vi "OCTavion_ScanControl_Host.vi"() -> ()   [LabVIEW 2016]
uses:
  <vilib>/FPGAPlugInAG/PCIe-7851R/niLvFpga_Open_PCIe-7851R.vi
  <vilib>/rvi/interface/common/dynamic/niFpgaDynamicAddResources.vi
  <vilib>/Utility/error.llb/Error Cluster From Error Code.vi
  <vilib>/rvi/errors/niLvFpgaAdjustHostInterfaceError.vi
  <vilib>/FPGAPlugInAG/Dynamic/niLvFpga_Close_Dynamic.vi
  <vilib>/rvi/interface/nirviOpenFPGA/nirviOpenFPGA.xnode
  FPGA/FPGA Bitfiles/OCTavionScanCont_FPGATarget_OCTavionScanCont_mQLUXe6JE5s.lvbitx
  <vilib>/rvi/interface/nirviReadWriteControl/nirviReadWriteControl.xnode
  <vilib>/rvi/interface/nirviCloseFPGA/nirviCloseFPGA.xnode
  NiFpgaLv.dll
  <vilib>/rvi/interface/Simulation/niFpgaSimulationCallBeginRW.vi
panel:
  in  "ScanParameters":T1
  out "FPGA output":T2
  in  "Stop":bool
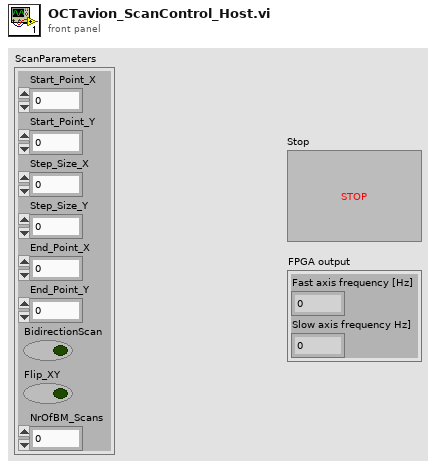
[diagram p1: front panel]
types:
  T1 = cluster{"Start_Point_X":i16, "Start_Point_Y":i16, "Step_Size_X":i16, "Step_Size_Y":i16, "End_Point_X":i16, "End_Point_Y":i16, "BidirectionScan":bool, "Flip_XY":bool, "NrOfBM_Scans":u16}
  T2 = cluster{"Fast axis frequency [Hz]":i16, "Slow axis frequency Hz]":i16}
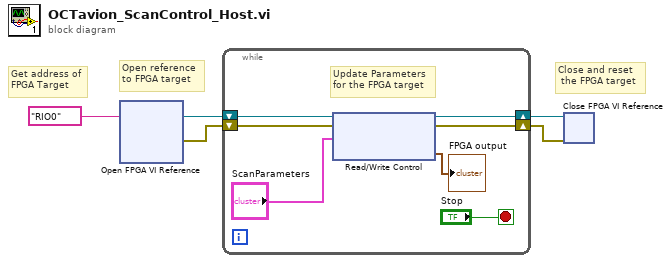
[diagram p0: block diagram]
diagram:
  # "Close and reset\n the FPGA target"
  # "Open reference\nto FPGA target"
  # "Get address of\nFPGA Target"
  n1 = xnode "Open FPGA VI Reference"("resource name"=tag "RIO0") -> ("FPGA VI Reference Out"=w4:refnum<k20>, "error out"=w2:errorcluster)  [unwired: 1 in]
  n2 = while {
    shift-right: [w11] -> w3
    shift-left: w4 -> [w12]
    shift-right: [w9] -> w1
    shift-left: w2 -> [w10]
    stop <- "Stop" stop-if-true
    # "Update Parameters\nfor the FPGA target"
    n3 = xnode "Read/Write Control"("FPGA VI Reference In"=w12, "error in"=w10, "ScanParameters"="ScanParameters") -> ("FPGA VI Reference Out"=w11:refnum<k20>, "error out"=w9:errorcluster, "FPGA output"=→"FPGA output":T2)
  }
  n4 = xnode "Close FPGA VI Reference"("FPGA VI Reference In"=w3, "error in"=w1) -> ()  [unwired: 1 out]
